vi "WK6425_CommandsGlobal.vi"() -> ()   [LabVIEW 2013, in "WK6425.lvclass"]
uses:
  WK6425.lvclass
panel:
  in  "WayneKerr 6425 GPIB Setup":T1={"GPIB address"="17", "Instrument name"="WayneKerr 6425", "Instrument type"=1, "Command \"Initialise LCR\""="%s;FREQ%d;LEV%1.2fV;AUT;NORS;C;TRG", "Command \"OC Trim\""="TOC", "Command \"LCR Readout\""="TRG"} {"Instrument type" items=["Supply", "LCR"]}
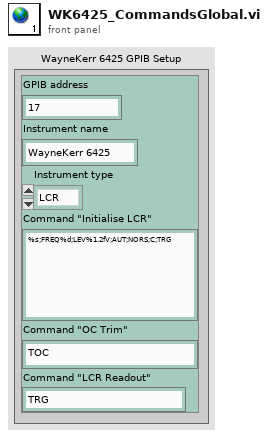
[diagram p1: front panel]
types:
  T1 = cluster{"GPIB address":string, "Instrument name":string, "Instrument type":u16, "Command \"Initialise LCR\"":string, "Command \"OC Trim\"":string, "Command \"LCR Readout\"":string}
diagram:
